vi "Inc.vi"(8 "error in (no error)":errorcluster, 9 "taskId":i32(ring) items=["TLibrary", "T01", "T02", "T03", "T04", "T05", "T06", "T07", "T08", "T09", "T10", "T11", "T12", "T13", "T14", "T15", "T16", "T17", "T18", "T19", "T20", "T21", "T22", "T23", "T24", "T25", "T26", "T27", "T28", "T29", "T30", "T31"], 11 "controller in":refnum<k24>) -> (0 "error out":errorcluster, 3 "controller out":refnum<k24>)   [LabVIEW 2016, in "Aerotech VIs.lvlib"]
uses:
  Aerotech VIs.lvlib
  C:/Program Files (x86)/Aerotech/A3200/LabVIEW/2010/Bin/Aerotech.A3200.dll
  C:/Program Files (x86)/Aerotech/A3200/LabVIEW/2010/Bin/Aerotech.A3200.LabVIEW.dll
panel:
  in  "return immediately":bool
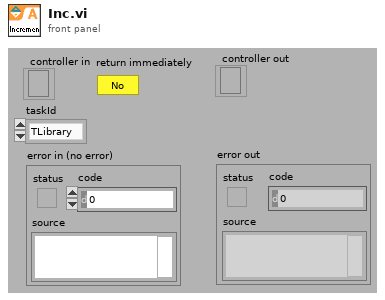
[diagram p1: front panel]
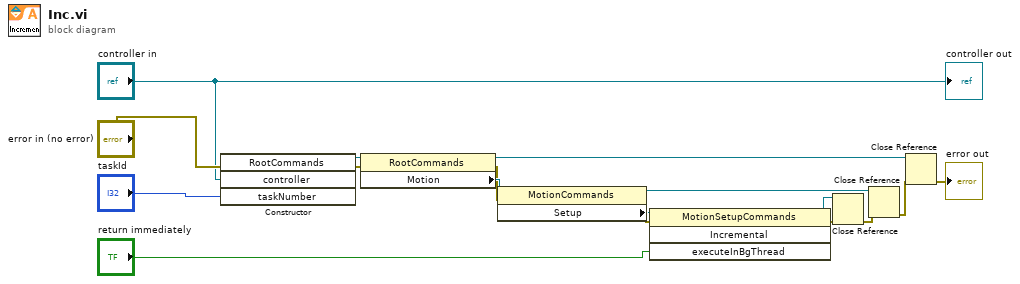
[diagram p0: block diagram]
diagram:
  n1 = constructor class="RootCommands"(error in="error in (no error)", "controller"="controller in", "taskNumber"="taskId") -> (reference out=w13:refnum<k24>, error out=w12:errorcluster)  [unwired: 2 in, 3 out]
  n2 = property class="RootCommands"(reference=w13, error in=w12) -> (reference out=w2:refnum<k24>, error out=w10:errorcluster, "Motion"=w11:refnum<k24>)
  n3 = property class="MotionCommands"(reference=w11, error in=w10) -> (reference out=w9:refnum<k24>, error out=w8:errorcluster, "Setup"=w7:refnum<k24>)
  n4 = invoke class="MotionSetupCommands" method="Incremental"(reference=w7, error in=w8, "executeInBgThread"="return immediately") -> (reference out=w16:refnum<k24>, error out=w17:errorcluster)  [unwired: 1 in, 2 out]
  n5 = Close Reference(reference=w16, error in (no error)=w17) -> (error out=w15:errorcluster)
  n6 = Close Reference(reference=w9, error in (no error)=w15) -> (error out=w1:errorcluster)
  n7 = Close Reference(reference=w2, error in (no error)=w1) -> (error out=→"error out":errorcluster)
  "controller out" <- "controller in"
